vi "Calculate Result (SubVI).vi"(8 "error in":errorcluster, 10 "Stored Values":dbl[](array[numeric]), 11 "Operator Array":T1[](array[typedef])) -> (0 "error out":errorcluster, 3 "Result":dbl)   [LabVIEW 2021]
doc: "Performs the mathematical operations (add, subtract, multiply and divide) in sequence and returns the final result."
uses:
  Controls/Operator Types.ctl
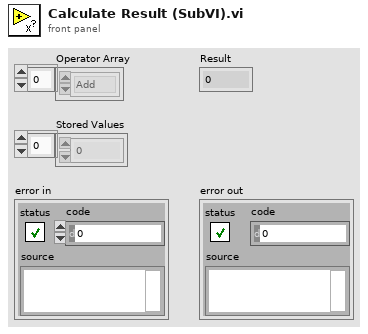
[diagram p1: front panel]
types:
  T1 = typedef "Operator Types.ctl" = enum16{"Add", "Subtract", "Multiply", "Divide"}
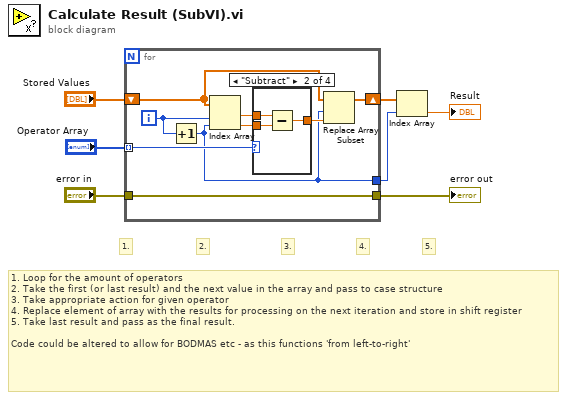
[diagram p0: block diagram]
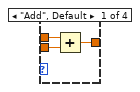
[diagram p2: hidden frame]
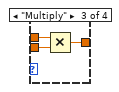
[diagram p3: hidden frame]
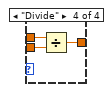
[diagram p4: hidden frame]
diagram:
  # "5."
  # "4."
  # "3."
  # "2."
  # "1. Loop for the amount of operators\n2. Take the first (or last result) and the next value in the array and pass to case structure\n3. Take appropriate action for given operator\n4. Replace element of array with the results for processing on the next iteration and store in shift register\n5. Take last result and pass as the final result.\n\nCode could be altered to allow for BODMAS etc - as this functions 'from left-to-right'"
  # "1."
  n1 = for {
    tunnel: "error in" -> [w9]
    tunnel: "Operator Array" -> [w15] mode=indexing
    shift-right: [w10] -> w4
    shift-left: "Stored Values" -> [w11]
    tunnel: [w9] -> w5
    tunnel: [w8] -> w7
    i -> [w16]
    n2 = Increment(x=w16) -> (x+1=w8:i32)
    n3 = Index Array(array=w11, index #1=w16, index #2=w8) -> (element #1=w14:dbl, element #2=w13:dbl)
    n4 = case shown="\"Subtract\"" w15 {
      tunnel: w14 -> [w19 w22 w25 w27]
      tunnel: w13 -> [w18 w21 w24 w28]
      tunnel: [w17 w20 w23 w26] -> w12
      frame "Add", Default {
        n5 = Add(x=w19, y=w18) -> (x+y=w17:dbl)
      }
      frame "Subtract" {
        n6 = Subtract(x=w22, y=w21) -> (x-y=w20:dbl)
      }
      frame "Multiply" {
        n7 = Multiply(x=w25, y=w24) -> (x*y=w23:dbl)
      }
      frame "Divide" {
        n8 = Divide(x=w27, y=w28) -> (x/y=w26:dbl)
      }
    }
    n9 = Replace Array Subset(array=w11, new element=w12, index=w8) -> (w10:dbl[])
  }
  "error out" <- w5
  n10 = Index Array(array=w4, index=w7) -> (element=→"Result":dbl)
